vi "Test Deserialize Signed Integers.vi"(8 "error in (no error)":errorcluster) -> (0 "error out":errorcluster)   [LabVIEW 2013]
uses:
  src/Serializer/JSON Serializer/JSON Serializer.lvclass
  src/Deserializer/JSON Deserializer/JSON Deserializer.lvclass
  <vilib>/addons/_JKI Toolkits/Caraya/classes/Test/Test.lvclass
  <vilib>/addons/_JKI Toolkits/Caraya/classes/Assert/Assert.lvclass
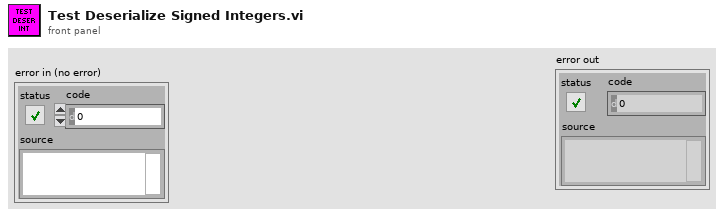
[diagram p1: front panel]
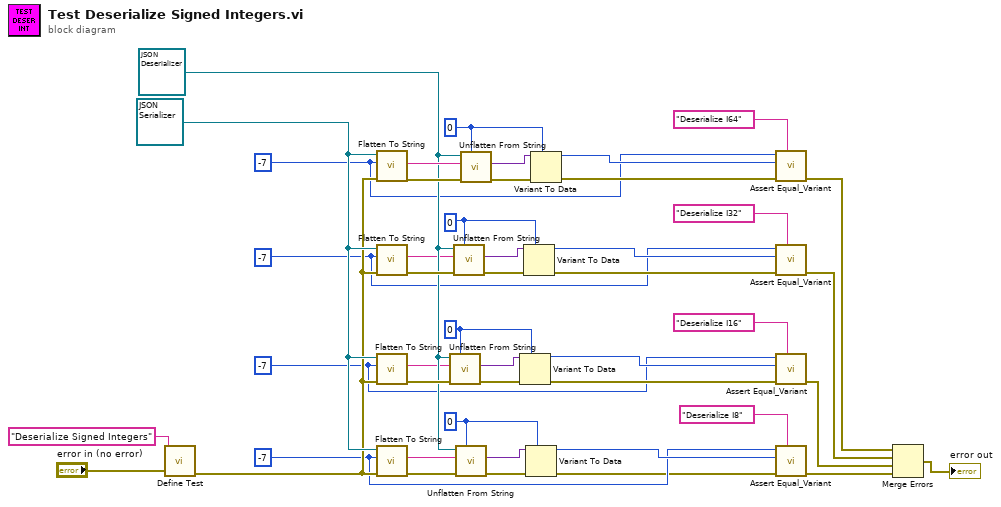
[diagram p0: block diagram]
diagram:
  w2 = i64 0
  w3 = 0
  w4 = i16 0
  w5 = i8 0
  w18 = refnum<class "JSON Deserializer.lvclass"> refnum ("Deserializer in")
  w41 = refnum<class "JSON Serializer.lvclass"> refnum ("JKI JSON Serialization.lvlib:JSON Serializer.lvclass")
  w6 = i8 -7
  w9 = i64 -7
  w7 = i16 -7
  w8 = -7
  n1 = call <vilib>:"Define Test.vi"("error in (no error)"="error in (no error)", "Label (VI Title)"="Deserialize Signed Integers") -> ("error out"=w40:errorcluster)  [unwired: 9 in]
  n2 = call-dynamic "Flatten To String.vi"("error in (no error)"=w40, "Variant"=w9, "JSON Serializer in"=w41) -> ("error out"=w33:errorcluster, "String"=w32:string)  [unwired: 6 in, 1 out]
  n3 = call-dynamic "Flatten To String.vi"("error in (no error)"=w40, "Variant"=w8, "JSON Serializer in"=w41) -> ("error out"=w19:errorcluster, "String"=w15:string)  [unwired: 6 in, 1 out]
  n4 = call-dynamic "Flatten To String.vi"("error in (no error)"=w40, "Variant"=w7, "JSON Serializer in"=w41) -> ("error out"=w20:errorcluster, "String"=w17:string)  [unwired: 6 in, 1 out]
  n5 = call-dynamic "Flatten To String.vi"("error in (no error)"=w40, "Variant"=w6, "JSON Serializer in"=w41) -> ("error out"=w21:errorcluster, "String"=w16:string)  [unwired: 6 in, 1 out]
  n6 = call-dynamic "Unflatten From String.vi"("Type and Defaults"=w4, "error in (no error)"=w20, "String"=w17, "Deserializer in"=w18) -> ("error out"=w23:errorcluster, "Variant"=w22:variant)  [unwired: 5 in, 1 out]
  n7 = call-dynamic "Unflatten From String.vi"("Type and Defaults"=w3, "error in (no error)"=w19, "String"=w15, "Deserializer in"=w18) -> ("error out"=w27:errorcluster, "Variant"=w26:variant)  [unwired: 5 in, 1 out]
  n8 = call-dynamic "Unflatten From String.vi"("Type and Defaults"=w5, "error in (no error)"=w21, "String"=w16, "Deserializer in"=w18) -> ("error out"=w25:errorcluster, "Variant"=w24:variant)  [unwired: 5 in, 1 out]
  n9 = call-dynamic "Unflatten From String.vi"("Type and Defaults"=w2, "error in (no error)"=w33, "String"=w32, "Deserializer in"=w18) -> ("error out"=w31:errorcluster, "Variant"=w30:variant)  [unwired: 5 in, 1 out]
  n10 = Variant To Data(error in=w23, type=w4, Variant=w22) -> (data=w12:i16, error out=w13:errorcluster)
  n11 = Variant To Data(error in=w27, type=w3, Variant=w26) -> (data=w10:i32, error out=w14:errorcluster)
  n12 = Variant To Data(error in=w25, type=w5, Variant=w24) -> (data=w11:i8, error out=w1:errorcluster)
  n13 = Variant To Data(error in=w31, type=w2, Variant=w30) -> (data=w29:i64, error out=w28:errorcluster)
  n14 = call <vilib>:"Assert Equal_Variant.vi"("Label"="Deserialize I64", "error in (no error)"=w28, "Y"=w29, "X"=w9) -> ("error out"=w35:errorcluster)  [unwired: 7 in]
  n15 = call <vilib>:"Assert Equal_Variant.vi"("Label"="Deserialize I32", "error in (no error)"=w14, "Y"=w10, "X"=w8) -> ("error out"=w36:errorcluster)  [unwired: 7 in]
  n16 = call <vilib>:"Assert Equal_Variant.vi"("Label"="Deserialize I16", "error in (no error)"=w13, "Y"=w12, "X"=w7) -> ("error out"=w37:errorcluster)  [unwired: 7 in]
  n17 = call <vilib>:"Assert Equal_Variant.vi"("Label"="Deserialize I8", "error in (no error)"=w1, "Y"=w11, "X"=w6) -> ("error out"=w38:errorcluster)  [unwired: 7 in]
  n18 = Merge Errors(w35, w36, w37, w38) -> (→"error out":errorcluster)
